vi "Square Preserve Sign.vi"(1 "In":dbl) -> (0 "Out":dbl)   [LabVIEW 2012]
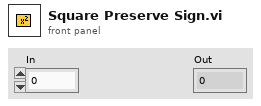
[diagram p1: front panel]
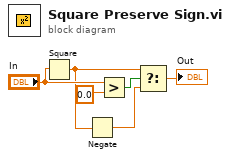
[diagram p0: block diagram]
diagram:
  n1 = Square(x="In") -> (x^2=w3:dbl)
  n2 = Negate(x=w3) -> (-x=w2:dbl)
  n3 = Greater?(x="In", y=0.0) -> (0:w5:bool)
  n4 = Select(t=w3, s=w5, f=w2) -> (s? t:f=→"Out":dbl)
